vi "Single Calculate Function Query.vi"(8 "error in":errorcluster, 10 "Calculation Channel":i32(ring) items=["Calc Channel 1", "Calc Channel 2", "Calc Channel 3", "Calc Channel 4"], 11 "Instrument Handle In":i32) -> (0 "error out":errorcluster, 1 "Operation":i32(ring) items=["Add", "Absolute Value", "Copy", "Derivative", "Integrate", "Invert", "Multiply", "Subtract", "Limit Test", "FFT", "Smooth", "Measurement", "Histogram", "No Operation"], 3 "Instrument Handle Out":i32, 4 "Source2":i32(ring) caption="Source 2" items=["Input Channel 1", "Input Channel 2", "Input Channel 3", "Input Channel 4", "Calc Channel 1", "Calc Channel 2", "Calc Channel 3", "Calc Channel 4", "Ref Channel 1", "Ref Channel 2", "Ref Channel 3", "Ref Channel 4"], 5 "Source1":i32(ring) caption="Source 1" items=["Input Channel 1", "Input Channel 2", "Input Channel 3", "Input Channel 4", "Calc Channel 1", "Calc Channel 2", "Calc Channel 3", "Calc Channel 4", "Ref Channel 1", "Ref Channel 2", "Ref Channel 3", "Ref Channel 4"])   [LabVIEW 8.6, in "ZTScopeM.lvlib"]
doc: "Query the configuration of the selected calculation channel."
uses:
  ZTScopeM.lvlib
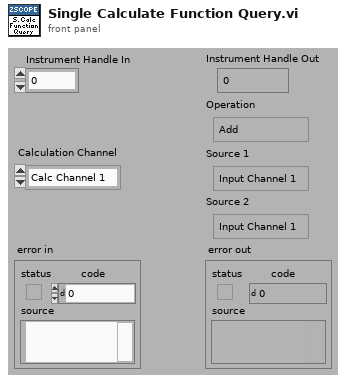
[diagram p1: front panel]
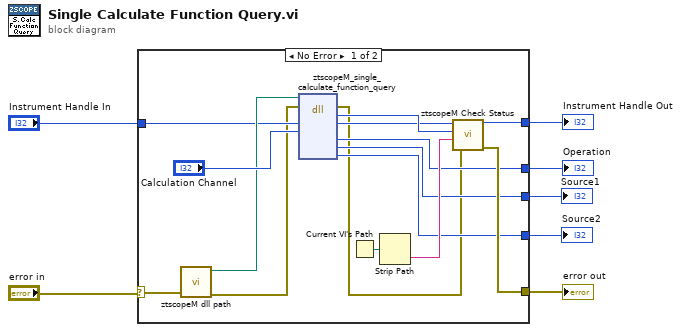
[diagram p0: block diagram]
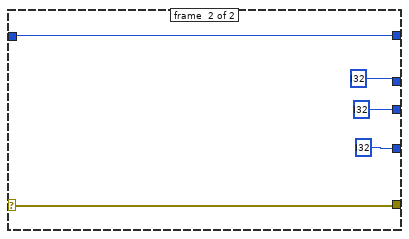
[diagram p2: hidden frame]
diagram:
  n1 = case shown="No Error" "error in" {
    selector: "error in" -> [w12 w27]
    tunnel: [w17 w27] -> w6
    tunnel: [w18 w23] -> w5
    tunnel: [w15 i32 ? ("instrumentHandle")] -> w4
    tunnel: [w14 i32 ? ("instrumentHandle")] -> w3
    tunnel: [w13 i32 ? ("instrumentHandle")] -> w2
    tunnel: "Instrument Handle In" -> [w10 w23]
    frame #0 {
      n2 = call "ztscopeM dll path.vi"("error in (no error)"=w12) -> ("error out"=w9:errorcluster, "<instrument>.dll path"=w11:path)  [unwired: 9 in]
      n3 = dll-call lib="C:/Program Files (x86)/National Instruments/LabVIEW 2013/instr.lib/ztscopem/ztscopeM.dll" fn="ztscopeM_single_calculate_function_query"(path in=w11, error in=w9, "instrumentHandle"=w10, "calculationChannel"="Calculation Channel") -> (error out=w8:errorcluster, w22:i32, "instrumentHandle"=w21:i32, "operation"=w15:i32, "source1"=w14:i32, "source2"=w13:i32)  [unwired: 2 in, 4 out]
      n4 = Current VI's Path() -> (path=w20:path)
      n5 = Strip Path(path=w20) -> (name=w19:string)  [unwired: 1 out]
      n6 = call "ztscopeM Check Status.vi"("error in"=w8, "name of VI"=w19, "status (return code)"=w22, "instrument handle in"=w21) -> ("error out"=w17:errorcluster, "instrument handle out"=w18:i32)  [unwired: 2 out]
    }
    frame #1 {
    }
  }
  "Instrument Handle Out" <- w5
  "error out" <- w6
  "Operation" <- w4
  "Source1" <- w3
  "Source2" <- w2
